vi "Apply Endpoint Configuration.vi"(8 "error in (no error)":errorcluster, 9 "Endpoint":string, 10 "Endpoint Config Section Ref in":T2 format="%.0x", 11 "Refnum in":T1) -> (0 "error out":errorcluster, 1 "Endpoint Addressable?":bool, 2 "Endpoint Configuration Section Ref out":T2 format="%.0x", 3 "Refnum out":T1)   [LabVIEW 2017, in "SLSC Switch Scripting.lvlib"]
uses:
  SLSC Switch Scripting.lvlib
  <vilib>/NI Veristand/Custom Device API/Custom Device Item Ref.ctl
  <vilib>/userdefined/High Color/SLSC_Switch/nislscslSession.ctl
  <resource>/objmgr/nislscsl.rc
  <vilib>/NI Veristand/Custom Device API/Custom Device API.lvlib
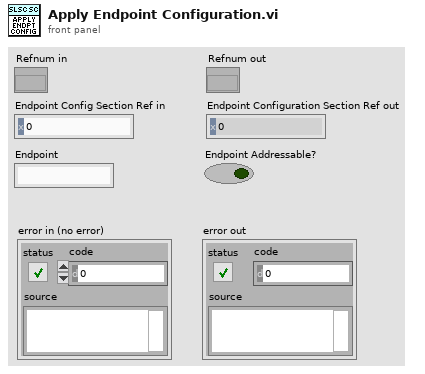
[diagram p1: front panel]
types:
  T1 = typedef "nislscslSession.ctl" = refnum<k20>
  T2 = typedef "Custom Device API.lvlib/Custom Device Item Ref.ctl" = u64
  T3 = typedef "SLSC Switch Shared.lvlib/Endpoint Configuration Enum.ctl" = enum16{"Load", "Source", "Configuration"}
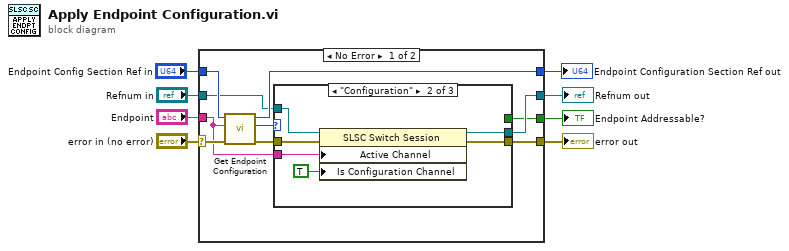
[diagram p0: block diagram]
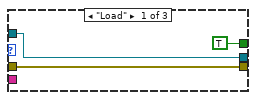
[diagram p2: hidden frame]
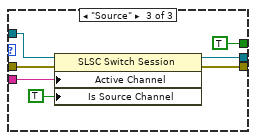
[diagram p3: hidden frame]
diagram:
  n1 = case shown="No Error" "error in (no error)" {
    selector: "error in (no error)" -> [w14 w37]
    tunnel: [w18 w35] -> w8
    tunnel: [w17 w37] -> w7
    tunnel: [w15 w36] -> w6
    tunnel: "Endpoint Config Section Ref in" -> [w13 w35]
    tunnel: "Endpoint" -> [w12 _]
    tunnel: [w10 _] -> w2
    tunnel: "Refnum in" -> [w9 w36]
    frame No Error {
      n2 = call "Get Endpoint Configuration.vi"("error in (no error)"=w14, "Endpoint"=w12, "Endpoint Configuration Section Ref in"=w13) -> ("error out"=w16:errorcluster, "Configuration Type"=w11:T3, "Endpoint Configuration Section Ref out"=w18:T2)  [unwired: 6 in]
      n3 = case shown="\"Configuration\"" w11 {
        tunnel: w9 -> [w20 w26 w34]
        tunnel: w12 -> [_ w27 w32]
        tunnel: [TRUE _ TRUE] -> w10
        tunnel: [w20 w24 w30] -> w15
        tunnel: w16 -> [w19 w23 w28]
        tunnel: [w19 w22 w29] -> w17
        frame "Load" {
        }
        frame "Configuration" {
          n4 = property class="SLSC Switch Session"(reference=w26, error in=w23, "Active Channel"=w27, "Is Configuration Channel"=TRUE ("Channel Configuration:Is Configuration Channel")) -> (reference out=w24:T1, error out=w22:errorcluster)
        }
        frame "Source" {
          n5 = property class="SLSC Switch Session"(reference=w34, error in=w28, "Active Channel"=w32, "Is Source Channel"=TRUE ("Channel Configuration:Is Source Channel")) -> (reference out=w30:T1, error out=w29:errorcluster)
        }
      }
    }
    frame Error {
    }
  }
  "Endpoint Configuration Section Ref out" <- w8
  "error out" <- w7
  "Refnum out" <- w6
  "Endpoint Addressable?" <- w2
